vi "UTIL Temp Control v2.vi"(4 "Evaluate":bool, 5 "Parameters In":dbl[](array[numeric]), 6 "Sleep Wake Ratio":dbl) -> (1 "Parameters Out":dbl[](array[numeric]), 3 "Q":dbl)   [LabVIEW 2010]
doc: "This VI keeps track of the number of Sleep and Wake classifications over a desired interval, and modifies the target ambient temperature based on the sleep-wake ratio. It stores 5 values in a shift register (Parameters In/Out):\n1. Error (Q - Q*)\n2. Target Temperature\n3. Sleep Count\n4. Wake Count\n5. Previous Temperature Change\n\nInputs: \n Class SGL, predicted sleep stage\n Parameters In 1-D Array of Double\n Evaluate Boolean, true at end of time period\nOutputs:\n Parameters Out 1-D Array of DBL"
uses:
  <vilib>/ptbypt/NI_PtbyPt.lvlib
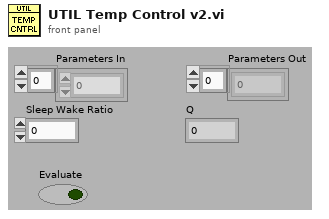
[diagram p1: front panel]
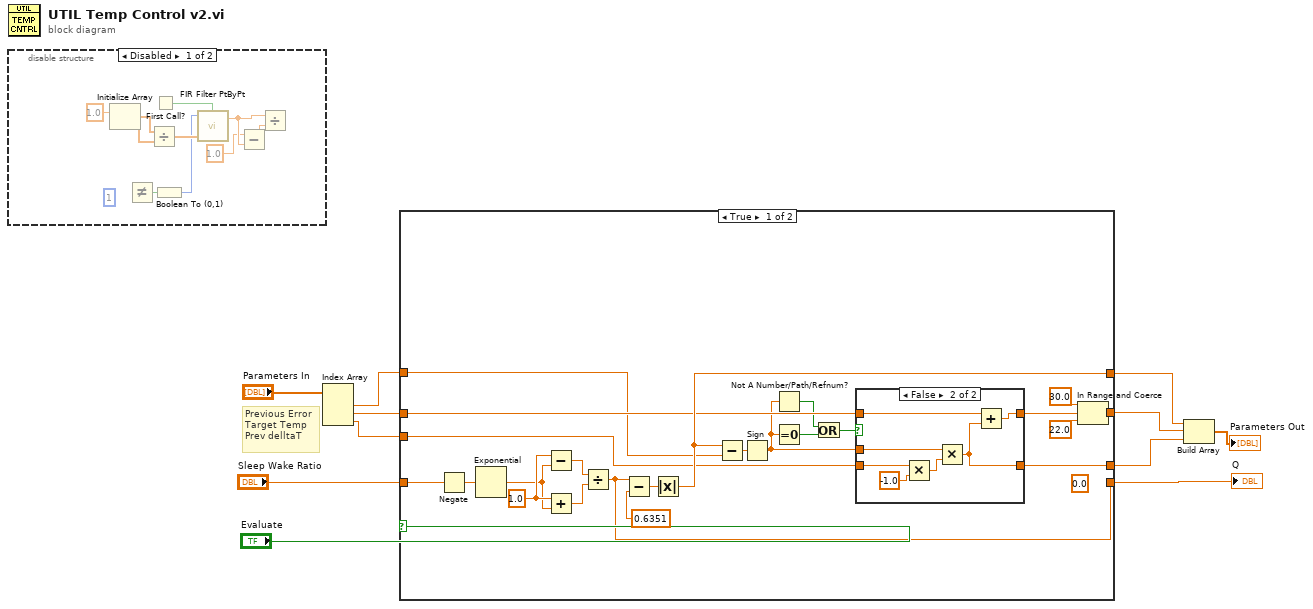
[diagram p0: block diagram]
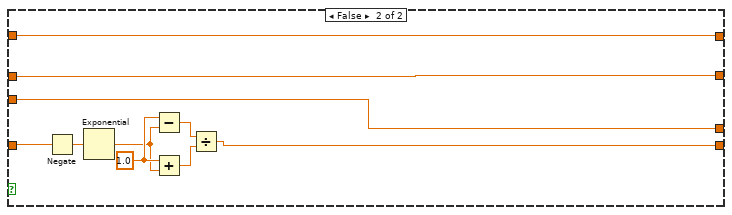
[diagram p4: hidden frame]
diagram:
  # "Previous Error\nTarget Temp\nPrev delltaT"
  n1 = disable-structure shown="Disabled" {
    frame Disabled {
      (unwired) 1 ("y")
      n2 = Not Equal?() -> (x != y?=w17:bool)  [unwired: 2 in]
      n3 = First Call?() -> (First Call?: T/F=w18:bool)
      n4 = Boolean To (0,1)(Boolean=w17) -> (0, 1=w16:i16)
      n5 = Initialize Array(1.0 ("element"), w12) -> (w20:dbl[])
      n6 = Divide(x=w20) -> (y=w12:dbl[], x/y=w19:dbl[])
      n7 = call <vilib>:"FIR Filter PtByPt.vi"("initialize"=w18, "Forward Coefficients"=w19, "x"=w16) -> ("Filtered x"=w15:dbl)  [unwired: 1 in, 1 out]
      n8 = Subtract(x=1.0 ("element"), y=w15) -> (x-y=w13:dbl)
      n9 = Divide(x=w15, y=w13) -> ()  [unwired: 1 out]
    }
    frame Enabled {
    }
  }
  n10 = Index Array(array="Parameters In") -> (element #1=w6:dbl, element #2=w5:dbl, element #3=w4:dbl)  [unwired: 3 in]
  n11 = case shown="True" "Evaluate" {
    tunnel: w6 -> [w35 w63]
    tunnel: [w40 w63] -> w10
    tunnel: [w42 w62] -> w9
    tunnel: w5 -> [w38 w62]
    tunnel: [w39 w61] -> w3
    tunnel: w4 -> [w36 w61]
    tunnel: [w23 w54] -> w2
    tunnel: "Sleep Wake Ratio" -> [w22 w55]
    frame True {
      w28 = 1.0 ("x")
      (unwired) 0.0
      n12 = Negate(x=w22) -> (-x=w27:dbl)
      n13 = Exponential(1:w27) -> (0:w26:dbl)
      n14 = Subtract(x=w28, y=w26) -> (x-y=w25:dbl)
      n15 = Add(x=w28, y=w26) -> (x+y=w24:dbl)
      n16 = Divide(x=w25, y=w24) -> (x/y=w23:dbl)
      n17 = Subtract(x=w23, y=0.6351) -> (x-y=w33:dbl)
      n18 = Absolute Value(x=w33) -> (abs(x)=w40:dbl)
      n19 = Subtract(x=w40, y=w35) -> (x-y=w41:dbl)
      n20 = Sign(1:w41) -> (0:w32:dbl)
      n21 = Not A Number/Path/Refnum?(number/path/refnum=w32) -> (NaN/Path/Refnum?=w29:bool)
      n22 = Equal To 0?(x=w32) -> (x = 0?=w31:bool)
      n23 = Or(x=w29, y=w31) -> (x .or. y?=w30:bool)
      n24 = case shown="False" w30 {
        tunnel: w36 -> [w45 w48]
        tunnel: [w45 w53] -> w39
        tunnel: w38 -> [w46 w52]
        tunnel: [w46 w51] -> w37
        tunnel: w32 -> [_ w50]
        frame True {
        }
        frame False {
          n25 = Multiply(x=w48, y=-1.0) -> (x*y=w47:dbl)
          n26 = Multiply(x=w50, y=w47) -> (x*y=w53:dbl)
          n27 = Add(x=w52, y=w53) -> (x+y=w51:dbl)
        }
      }
      n28 = In Range and Coerce(upper limit=30.0 ("element"), x=w37, lower limit=22.0 ("element")) -> (coerced(x)=w42:dbl)  [unwired: 1 out]
    }
    frame False {
      w60 = 1.0 ("x")
      n29 = Negate(x=w55) -> (-x=w59:dbl)
      n30 = Exponential(1:w59) -> (0:w58:dbl)
      n31 = Subtract(x=w60, y=w58) -> (x-y=w57:dbl)
      n32 = Add(x=w60, y=w58) -> (x+y=w56:dbl)
      n33 = Divide(x=w57, y=w56) -> (x/y=w54:dbl)
    }
  }
  "Q" <- w2
  n34 = Build Array(w10, w9, w3) -> (→"Parameters Out":dbl[])
